vi "Sample Command.vi"() -> (1 "Expected Response":string="ñò4Võ", 2 "Sample Command":string="ñò4Võ")   [LabVIEW 2017, in "Serial Device.lvclass"]
uses:
  Serial Device.lvclass
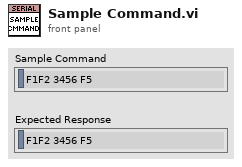
[diagram p1: front panel]
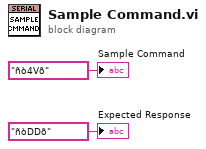
[diagram p0: block diagram]
diagram:
  "Sample Command" <- "ñò4Võ"
  "Expected Response" <- "ñòDDõ"
